vi "WOBOT NT Client.vi"(4 "Update Time":i32=100, 5 "Client Exit Notifier":refnum<notifier>, 9 "Client Name":string, 11 "Server IP Address":string="localhost") -> ()   [LabVIEW 2020]
doc: "Place this VI in the Dashboard or other client applications so that it can run in parallel with the other tasks. Provide the robot IP address so that it can know where to find the server.\n\nYou normally want the restart option to be true, but if you have your own restart strategy, you can disable it. Tracing is useful when debugging. Similarly, the disconnect timout may need to be raised if setting breakpoints. The user event ref will publish the client activities so that other elements of the dashboard are notified when packets are processed."
uses:
  NT Client States.ctl
  NT Client Cluster.ctl
  <vilib>/Rock Robotics/Network Tables/NT Event Type.ctl
  <vilib>/Rock Robotics/Network Tables/Protocol Operations.ctl
  <vilib>/Rock Robotics/Network Tables/Field Data.ctl
  <vilib>/Rock Robotics/Network Tables/Field Type.ctl
  <vilib>/Rock Robotics/Network Tables/Sequence.ctl
  <vilib>/Rock Robotics/Network Tables/Cnx List Operations.ctl
  <vilib>/Rock Robotics/Network Tables/NT Globals.vi
panel:
  in  "Tracing":bool
  out "Trace Strings":string
  in  "timeout":i32=1000
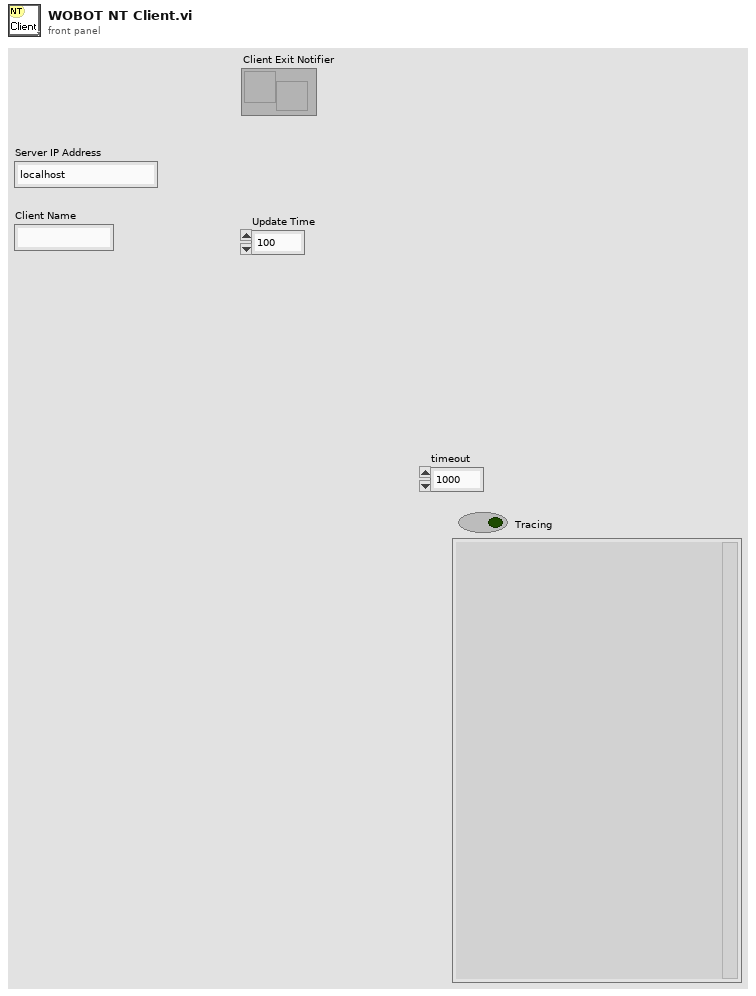
[diagram p1: front panel]
types:
  T1 = typedef "NT Client Cluster.ctl" = cluster{"connection ID":refnum<k5>, "error in":errorcluster, "Client Name":string, "Dirty notifier":refnum<notifier>, "Cancel notifier":refnum<notifier>, "Message":string, "Trace String":string, "user event ref":refnum<user-event>}
  T2 = typedef "NT Client States.ctl" = enum16{"Message Dispatcher", "INI", "TCP CLose", "TCP Read", "TCP Open", "TCP Write", "Exit"}
  T3 = typedef "Cnx List Operations.ctl" = enum16{"Add Cnx", "Remove Cnx", "Retrieve List", "Cnx Inited", "Check Cnx Name"}
  T4 = typedef "Event Setup Types.ctl" = enum16{"Default", "Camera Loop Started", "Save Data", "Open Front Panel", "Exit"}
  T5 = typedef "NT Event Type.ctl" = cluster{"Operation":T6, "Name":string, "Field Value":T7}
  T6 = typedef "Protocol Operations.ctl" = enum16{"Unknown", "Keep Alive", "Client Hello", "Version not supported", "Server Hello Complete", "Assign", "Update", "No Op", "Server Hello", "Client Hello Complete", "Update Flags", "Delete Entry", "Delete All", "RPC Exec", "RPC Response"}
  T7 = typedef "Field Data.ctl" = cluster{"Dbl":dbl, "String":string, "Type":T8, "Boolean":bool, "Sequence #":T9, "Flags":u8}
  T8 = typedef "Field Type.ctl" = enum8{"Invalid", "Bool", "Numeric", "String", "Raw", "Boolean Array", "Numeric Array", "String Array", "RPC"}
  T9 = typedef "Sequence.ctl" = u16
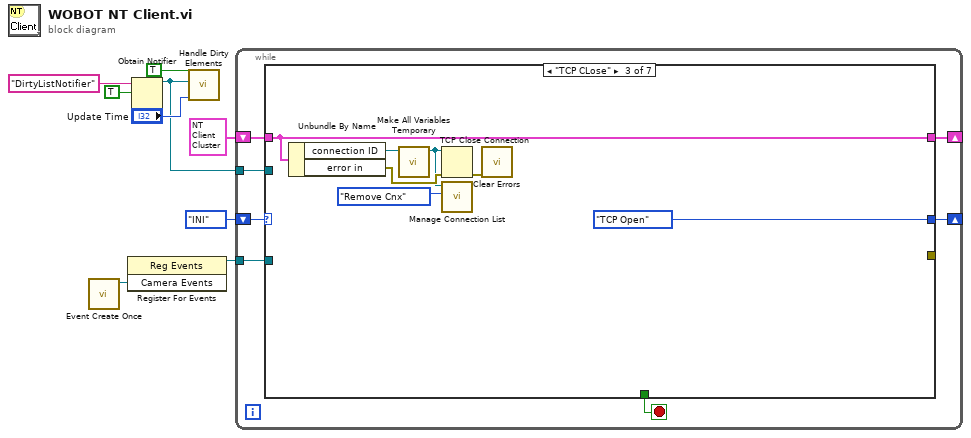
[diagram p0: block diagram]
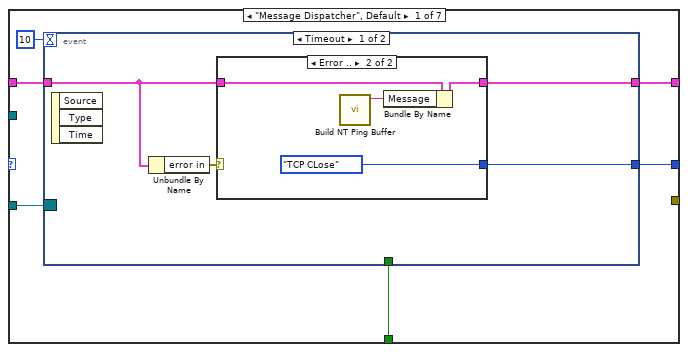
[diagram p2: hidden frame]
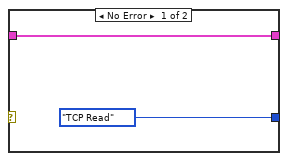
[diagram p3: hidden frame]
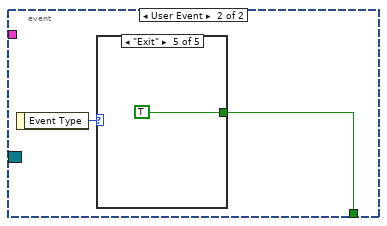
[diagram p4: hidden frame]
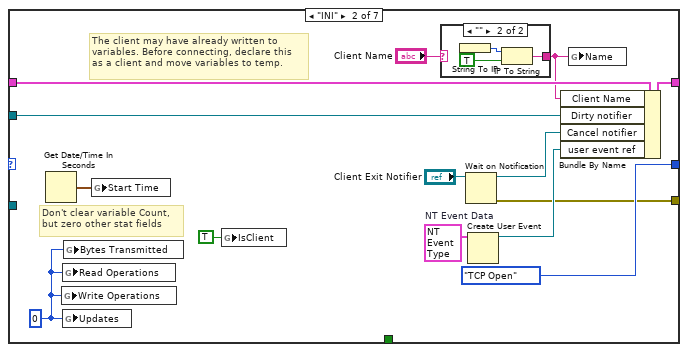
[diagram p9: hidden frame]
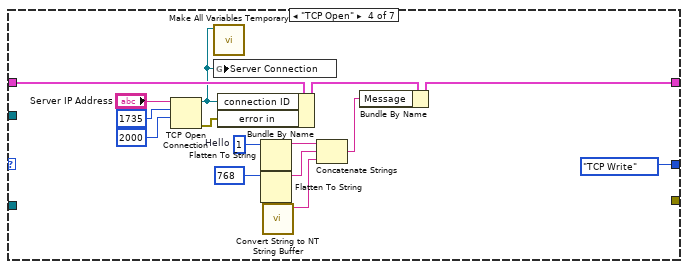
[diagram p11: hidden frame]
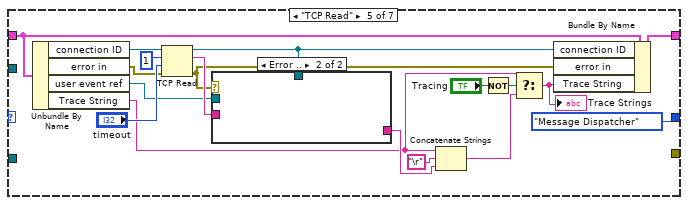
[diagram p12: hidden frame]
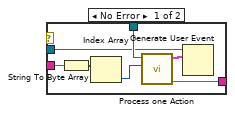
[diagram p13: hidden frame]
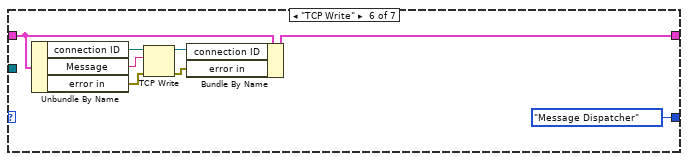
[diagram p14: hidden frame]
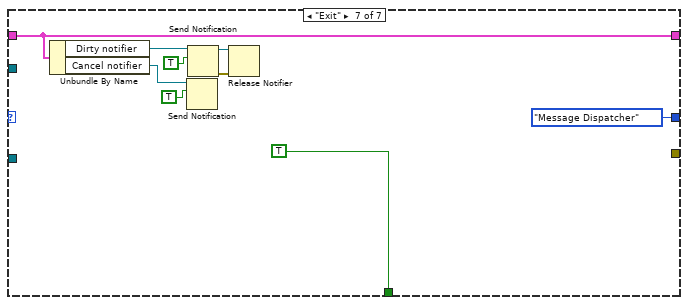
[diagram p15: hidden frame]
diagram:
  n1 = call "Event Create Once.vi"() -> ("Camera Events"=w7:refnum<user-event>)  [unwired: 10 in, 1 out]
  n2 = register-events(w7) -> (reference out=w6:refnum<event-registration>)  [unwired: 2 in, 1 out]
  n3 = Obtain Notifier(name (unnamed)="DirtyListNotifier", notification data type=TRUE ("IsClient")) -> (notifier out=w1:refnum<notifier>)  [unwired: 2 in, 2 out]
  n4 = call <vilib>:"Handle Dirty Elements.vi"("Update Time"="Update Time", "notifier out"=w1, "IsClient"=TRUE) -> ()  [unwired: 8 in, 1 out]
  n5 = while {
    shift-right: [w13] -> _
    shift-left: NT_Client_States."INI" -> [w16]
    shift-right: [w14] -> _
    shift-left: T1 {"connection ID"=refnum, "error in"={"status"=FALSE, "code"=0, "source"=""}, "Client Name"="", "Dirty notifier"=refnum, "Cancel notifier"=refnum, "Message"="", "Trace String"="", "user event ref"=refnum} -> [w15]
    tunnel: w6 -> [w12]
    tunnel: w1 -> [w10]
    stop <- w11 stop-if-true
    n6 = case shown="\"TCP CLose\"" w16 {
      tunnel: w15 -> [w20 w46 w60 w71 w90 w108 w115]
      tunnel: [w19 w45 w60 w65 w88 w104 w115] -> w14
      tunnel: [w22 NT_Client_States."TCP Open" NT_Client_States."TCP Open" NT_Client_States."TCP Write" NT_Client_States."Message Dispatcher" NT_Client_States."Message Dispatcher" NT_Client_States."Message Dispatcher"] -> w13
      tunnel: w12 -> [w18 _ _ _ _ _ _]
      tunnel: [w17 _ _ _ _ _ TRUE] -> w11
      tunnel: [_ w37 _ _ _ _ _] -> _
      tunnel: w10 -> [_ w36 _ _ _ _ _]
      frame "Message Dispatcher", Default {
        n7 = event shown="[0] Timeout" {
          selector: w18 -> [_ _]
          dyn-events: _ -> [_ _]
          timeout: 10 -> [_ _]
          tunnel: [w26 _] -> w22
          tunnel: w20 -> [w24 _]
          tunnel: [w23 _] -> w19
          tunnel: [_ w33] -> w17
          event Timeout {
            n8 = event-data() -> ()  [unwired: 1 in, 3 out]
            n9 = Unbundle By Name(w24) -> ("error in"=w25:errorcluster)
            n10 = case shown="Error .." w25 {
              tunnel: [NT_Client_States."TCP Read" NT_Client_States."TCP CLose"] -> w26
              tunnel: w24 -> [w27 w31]
              tunnel: [w27 w30] -> w23
              frame No Error {
              }
              frame Error {
                n11 = call <vilib>:"Build NT Ping Buffer.vi"() -> ("Data Buffer"=w29:string)  [unwired: 11 in]
                n12 = Bundle By Name(cluster=w31, "Message"=w29) -> (w30:T1)
              }
            }
          }
          event User Event {
            n13 = event-data() -> ("Event Type"=w34:T4)  [unwired: 1 in]
            n14 = case shown="\"Exit\"" w34 {
              tunnel: [_ _ _ _ TRUE] -> w33
              frame "Default", Default {
              }
              frame "Camera Loop Started" {
              }
              frame "Save Data" {
              }
              frame "Open Front Panel" {
              }
              frame "Exit" {
              }
            }
          }
        }
      }
      frame "INI" {
        w40 = T5 {"Operation"=enum."Assign", "Name"="", "Field Value"={"Dbl"=0.0, "String"="kjn", "Type"=enum."String", "Boolean"=FALSE, "Sequence #"=0, "Flags"=0}}  # NT Event Data
        w47 = 0 ("Updates")
        # "Don't clear variable Count,\nbut zero other stat fields"
        # "The client may have already written to\nvariables. Before connecting, declare this\nas a client and move variables to temp."
        n15 = Get Date/Time In Seconds() -> (seconds since 1Jan1904=w41:timestamp)
        n16 = global write "NT Globals.vi" "Write Operations"(w47) -> ()
        n17 = global write "NT Globals.vi" "Read Operations"(w47) -> ()
        n18 = global write "NT Globals.vi" "Updates"(w47) -> ()
        n19 = global write "NT Globals.vi" "Bytes Transmitted"(w47) -> ()
        n20 = global write "NT Globals.vi" "Start Time"(w41) -> ()
        n21 = global write "NT Globals.vi" "IsClient"(TRUE ("IsClient")) -> ()
        n22 = case shown="\"\"" "Client Name" {
          selector: "Client Name" -> [w50 _]
          tunnel: [w50 w51] -> w42
          frame Default {
          }
          frame "" {
            n23 = String To IP() -> (0:w53:u32)  [unwired: 1 in]
            n24 = IP To String(1:TRUE ("dot notation? (F)"), 2:w53) -> (0:w51:string)
          }
        }
        n25 = Wait on Notification(notifier="Client Exit Notifier") -> (notifier out=w44:refnum<notifier>, error out=w37:errorcluster)  [unwired: 3 in, 2 out]
        n26 = Create User Event(user event datatype=w40) -> (user event=w39:refnum<user-event>)  [unwired: 1 in, 1 out]
        n27 = Bundle By Name(cluster=w46, "Client Name"=w42, "Dirty notifier"=w36, "Cancel notifier"=w44, "user event ref"=w39) -> (w45:T1)
        n28 = global write "NT Globals.vi" "Name"(w42) -> ()
      }
      frame "TCP CLose" {
        n29 = Unbundle By Name(w60) -> ("connection ID"=w56:refnum<k5>, "error in"=w55:errorcluster)
        n30 = call <vilib>:"Make All Variables Temporary.vi"("connection ID"=w56) -> ("connection ID 2"=w54:refnum<k5>)  [unwired: 10 in]
        n31 = TCP Close Connection(connection ID=w54, error in (no error)=w55) -> (error out=w59:errorcluster)  [unwired: 1 in, 1 out]
        n32 = call <vilib>:"Manage Connection List.vi"("Operation"=Cnx_List_Operations."Remove Cnx", "connection ID"=w54) -> ()  [unwired: 5 in, 5 out]
        n33 = call <vilib>:"Clear Errors.vi"("error in (no error)"=w59) -> ()  [unwired: 5 in, 2 out]
      }
      frame "TCP Open" {
        w66 = u8 1  # Hello
        n34 = TCP Open Connection(address="Server IP Address", remote port or service name=u16 1735 ("port"), timeout ms (60000)=2000) -> (connection ID=w61:refnum<k5>, error out=w62:errorcluster)  [unwired: 2 in]
        n35 = call <vilib>:"Make All Variables Temporary.vi"("connection ID"=w61) -> ()  [unwired: 10 in, 1 out]
        n36 = global write "NT Globals.vi" "Server Connection"(w61) -> ()
        n37 = Bundle By Name(cluster=w71, "connection ID"=w61, "error in"=w62) -> (w72:T1)
        n38 = Flatten To String(anything=w66) -> (data string=w70:string)  [unwired: 3 in, 2 out]
        n39 = Flatten To String(anything=u16 768) -> (data string=w69:string)  [unwired: 3 in, 2 out]
        n40 = call <vilib>:"Convert String to NT String Buffer.vi"() -> ("NT Buffer"=w68:string)  [unwired: 11 in]
        n41 = Concatenate Strings(w70, w69, w68) -> (w64:string)
        n42 = Bundle By Name(cluster=w72, "Message"=w64) -> (w65:T1)
      }
      frame "TCP Read" {
        n43 = Unbundle By Name(w90) -> ("connection ID"=w89:refnum<k5>, "error in"=w86:errorcluster, "user event ref"=w77:refnum<user-event>, "Trace String"=w78:string)
        n44 = TCP Read(connection ID=w89, bytes to read=1 ("timeout ms (25000)"), error in (no error)=w86, 9:"timeout") -> (connection ID out=w87:refnum<k5>, data out=w91:string, error out=w84:errorcluster)  [unwired: 1 in]
        n45 = case shown="Error .." w84 {
          tunnel: w91 -> [w97 _]
          tunnel: w87 -> [w96 _]
          tunnel: [w95 _] -> w85
          tunnel: w77 -> [w94 _]
          frame No Error {
            n46 = String To Byte Array(string=w97) -> (unsigned byte array=w100:u8[])
            n47 = Index Array(array=w100) -> (element=w99:u8)  [unwired: 1 in]
            n48 = call <vilib>:"Process one Action.vi"("First Byte"=w99, "connection ID"=w96) -> ("Debug String"=w95:string, "NT Event Data"=w98:T5)  [unwired: 8 in]
            n49 = Generate User Event(user event=w94, event data cluster=w98) -> ()  [unwired: 2 in, 2 out]
          }
          frame Error {
          }
        }
        n50 = Concatenate Strings(w78, "\r", w85) -> (w79:string)
        n51 = Not(x="Tracing") -> (.not. x?=w80:bool)
        n52 = Select(t=w78, s=w80, f=w79) -> (s? t:f=w81:string)
        "Trace Strings" <- w81
        n53 = Bundle By Name(cluster=w90, "connection ID"=w87, "error in"=w84, "Trace String"=w81) -> (w88:T1)
      }
      frame "TCP Write" {
        n54 = Unbundle By Name(w108) -> ("connection ID"=w107:refnum<k5>, "Message"=w106:string, "error in"=w105:errorcluster)
        n55 = TCP Write(connection ID=w107, data in=w106, error in (no error)=w105) -> (connection ID out=w103:refnum<k5>, error out=w102:errorcluster)  [unwired: 1 in, 1 out]
        n56 = Bundle By Name(cluster=w108, "connection ID"=w103, "error in"=w102) -> (w104:T1)
      }
      frame "Exit" {
        n57 = Unbundle By Name(w115) -> ("Dirty notifier"=w114:refnum<notifier>, "Cancel notifier"=w111:refnum<notifier>)
        n58 = Send Notification(notification=TRUE, notifier=w111) -> ()  [unwired: 1 in, 2 out]
        n59 = Send Notification(notification=TRUE, notifier=w114) -> (notifier out=w117:refnum<notifier>, error out=w113:errorcluster)  [unwired: 1 in]
        n60 = Release Notifier(notifier=w117, error in (no error)=w113) -> ()  [unwired: 1 in, 3 out]
      }
    }
  }
